vi "getAttachmentPoint.vi"(0 "reference":refnum<class "SegmentedLineEdge.lvclass">, 1 "graphics":refnum<class "Graphics.lvclass">, 2 "p1":T1 {"y" format="%.2f"; "x" format="%.2f"}, 3 "p2":T1 {"y" format="%.2f"; "x" format="%.2f"}, 4 "text":string, 5 "error in (no error)":errorcluster, 7 "center":bool) -> (14 "reference out":refnum<class "SegmentedLineEdge.lvclass">, 15 "attachPoint":T1 {"y" format="%.2f"; "x" format="%.2f"}, 19 "error out":errorcluster)   [LabVIEW 2020, in "SegmentedLineEdge.lvclass"]
doc: "\"private static Point2D getAttachmentPoint(Graphics2D g2,"
uses:
  <resource>/Framework/Providers/Open_GDS/UML/SegmentedLineEdge_class/SegmentedLineEdge.lvclass
  <resource>/Framework/Providers/Open_GDS/UML/General/Point/Point Point2D.ctl
  <resource>/Framework/Providers/Open_GDS/UML/Graphics_class/Graphics.lvclass
  <resource>/Framework/Providers/Open_GDS/UML/General/Rectangle/Rectangle Rectangle2D.ctl
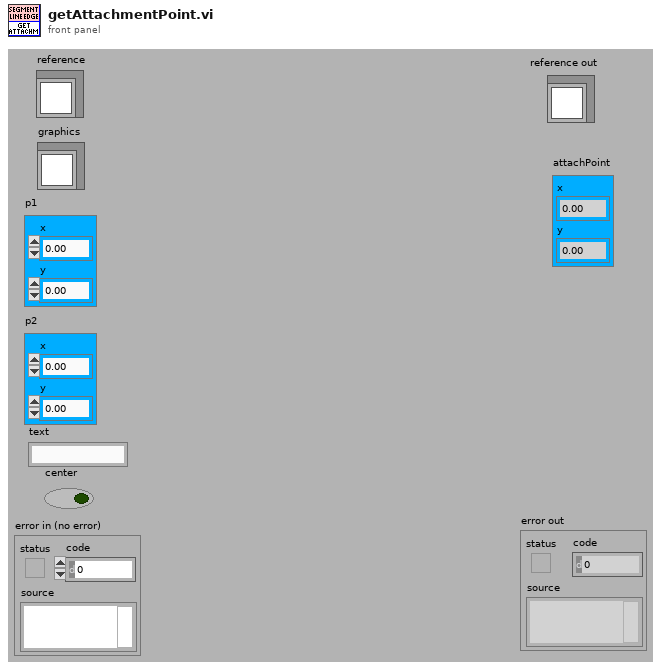
[diagram p1: front panel]
types:
  T1 = typedef "Point Point2D.ctl" = cluster{"x":dbl, "y":dbl}
  T2 = typedef "Rectangle Rectangle2D.ctl" = cluster{"x":dbl, "y":dbl, "width":dbl, "height":dbl}
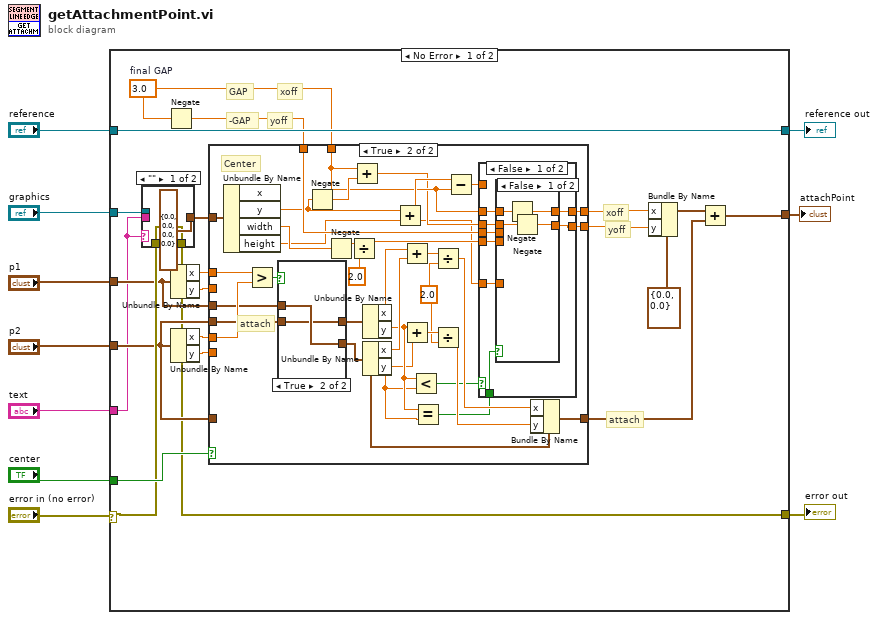
[diagram p0: block diagram]
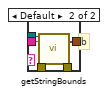
[diagram p2: hidden frame]
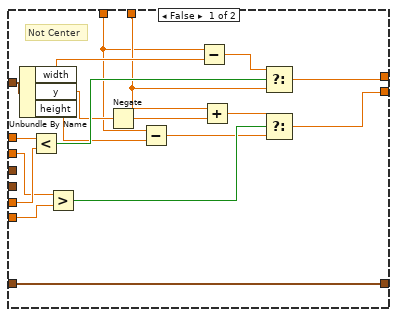
[diagram p3: hidden frame]
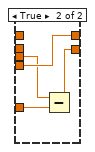
[diagram p4: hidden frame]
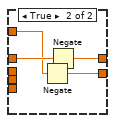
[diagram p5: hidden frame]
diagram:
  n1 = case shown="No Error" "error in (no error)" {
    selector: "error in (no error)" -> [w27 w116]
    tunnel: "reference" -> [w28 w117]
    tunnel: [w12 w116] -> w9
    tunnel: [w28 w117] -> w8
    tunnel: "graphics" -> [w31 _]
    tunnel: "text" -> [w11 _]
    tunnel: [w18 _] -> w4
    tunnel: "center" -> [w29 _]
    tunnel: "p1" -> [w24 _]
    tunnel: "p2" -> [w21 _]
    frame No Error {
      w23 = 3.0  # final GAP
      # "yoff"
      # "xoff"
      # "attach"
      # "yoff"
      # "xoff"
      # "GAP"
      # "-GAP"
      n2 = case shown="\"\"" w11 {
        tunnel: w31 -> [_ w38]
        tunnel: w11 -> [_ w37]
        tunnel: w27 -> [w32 w36]
        tunnel: [T2 {"x"=0.0, "y"=0.0, "width"=0.0, "height"=0.0} ("bounds") w35] -> w15
        tunnel: [w32 w34] -> w12
        frame "" {
        }
        frame Default {
          # "b"
          n3 = call-dynamic "getStringBounds.vi"("reference"=w38, "text"=w37, "error in (no error)"=w36) -> ("bounds"=w35:T2, "error out"=w34:errorcluster)  [unwired: 2 in, 13 out]
        }
      }
      n4 = Negate(x=w23) -> (-x=w22:dbl)
      n5 = Unbundle By Name(w24) -> ("x"=w26:dbl, "y"=w14:dbl)
      n6 = Unbundle By Name(w21) -> ("x"=w25:dbl, "y"=w13:dbl)
      n7 = case shown="True" w29 {
        tunnel: w26 -> [w57 w91]
        tunnel: w25 -> [w56 w90]
        tunnel: w24 -> [_ w88]
        tunnel: w21 -> [_ w87]
        tunnel: w22 -> [w41 w67]
        tunnel: w23 -> [w47 w60]
        tunnel: w21 -> [w55 _]
        tunnel: [w55 w79] -> w19
        tunnel: [w45 w74] -> w17
        tunnel: [w53 w68] -> w16
        tunnel: w15 -> [w52 w76]
        tunnel: w14 -> [w44 _]
        tunnel: w13 -> [w43 _]
        frame False {
          # "Not Center"
          n8 = Unbundle By Name(w52) -> ("width"=w51:dbl, "y"=w49:dbl, "height"=w39:dbl)
          n9 = Less?(x=w57, y=w56) -> (x < y?=w54:bool)
          n10 = Greater?(x=w44, y=w43) -> (0:w42:bool)
          n11 = Negate(x=w49) -> (-x=w48:dbl)
          n12 = Subtract(x=w41, y=w39) -> (x-y=w40:dbl)
          n13 = Subtract(x=w41, y=w51) -> (x-y=w50:dbl)
          n14 = Add(x=w47, y=w48) -> (x+y=w46:dbl)
          n15 = Select(t=w50, s=w54, f=w47) -> (s? t:f=w53:dbl)
          n16 = Select(t=w46, s=w42, f=w40) -> (s? t:f=w45:dbl)
        }
        frame True {
          w81 = 2.0 ("y")
          # "attach"
          # "Center"
          n17 = Unbundle By Name(w76) -> ("y"=w62:dbl, "width"=w65:dbl, "height"=w58:dbl)  [unwired: 1 out]
          n18 = Greater?(x=w91, y=w90) -> (0:w89:bool)
          n19 = case shown="True" w89 {
            tunnel: w88 -> [w113 w115]
            tunnel: [w112 w115] -> w80
            tunnel: [w113 w114] -> w86
            tunnel: w87 -> [w112 w114]
            frame False {
            }
            frame True {
            }
          }
          n20 = Negate(x=w62) -> (-x=w61:dbl)
          n21 = Negate(x=w65) -> (-x=w64:dbl)
          n22 = Divide(x=w64, y=2.0) -> (x/y=w63:dbl)
          n23 = Add(x=w60, y=w61) -> (x+y=w59:dbl)
          n24 = Unbundle By Name(w86) -> ("x"=w85:dbl, "y"=w71:dbl)
          n25 = Unbundle By Name(w80) -> ("x"=w84:dbl, "y"=w70:dbl)
          n26 = Add(x=w62, y=w58) -> (x+y=w75:dbl)
          n27 = Add(x=w85, y=w84) -> (x+y=w83:dbl)
          n28 = Add(x=w71, y=w70) -> (x+y=w82:dbl)
          n29 = Less?(x=w71, y=w70) -> (x < y?=w72:bool)
          n30 = Equal?(x=w71, y=w70) -> (x = y?=w69:bool)
          n31 = Divide(x=w83, y=w81) -> (x/y=w78:dbl)
          n32 = Divide(x=w82, y=w81) -> (x/y=w77:dbl)
          n33 = Subtract(x=w75, y=w60) -> (x-y=w73:dbl)
          n34 = case shown="False" w72 {
            tunnel: [w98 w109] -> w74
            tunnel: w73 -> [_ w110]
            tunnel: w69 -> [w99 _]
            tunnel: w60 -> [w94 w111]
            tunnel: [w96 w108] -> w68
            tunnel: w67 -> [w97 _]
            tunnel: w63 -> [w95 _]
            tunnel: w59 -> [w93 _]
            tunnel: w58 -> [w92 _]
            frame False {
              n35 = case shown="False" w99 {
                tunnel: [w101 w104] -> w98
                tunnel: w97 -> [_ w105]
                tunnel: [w100 w107] -> w96
                tunnel: w95 -> [_ w107]
                tunnel: w94 -> [w103 _]
                tunnel: w93 -> [w102 _]
                tunnel: w92 -> [_ w106]
                frame False {
                  n36 = Negate(x=w103) -> (-x=w100:dbl)
                  n37 = Negate(x=w102) -> (-x=w101:dbl)
                }
                frame True {
                  n38 = Subtract(x=w105, y=w106) -> (x-y=w104:dbl)
                }
              }
            }
            frame True {
              n39 = Negate(x=w110) -> (-x=w109:dbl)
              n40 = Negate(x=w111) -> (-x=w108:dbl)
            }
          }
          n41 = Bundle By Name(cluster=w80, "x"=w78, "y"=w77) -> (w79:T1)
        }
      }
      n42 = Bundle By Name(cluster=T1 {"x"=0.0, "y"=0.0} ("attachPoint"), "x"=w16, "y"=w17) -> (w20:T1)
      n43 = Add(x=w20, y=w19) -> (x+y=w18:T1)
    }
    frame Error {
    }
  }
  "reference out" <- w8
  "error out" <- w9
  "attachPoint" <- w4
